vi "PulserHandle.vi"() -> ()   [LabVIEW 2010]
panel:
  out "Pulser opened":bool
  in  "Pulser Handle":u32
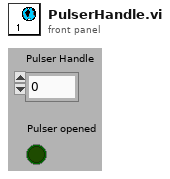
[diagram p1: front panel]
diagram:
